vi "Initialize.vi"(8 "error in":errorcluster, 9 "Timeout":u32=100 format="%.0f ms", 10 "Serial Settings":T1={"baud rate"=115200, "data bits"=8, "parity"=enum."None", "stop bits"=10, "flow control"=0} {"flow control" items=["None"=0, "XON/XOFF"=1, "RTS/CTS"=2, "DTR/DSR"=4]; "stop bits" items=["1.0"=10, "1.5"=15, "2.0"=20]; "data bits" min=5 max=8 step=1; "baud rate" items=["75"=75, "110"=110, "134"=134, "150"=150, "300"=300, "600"=600, "1200"=1200, "1800"=1800, "2400"=2400, "4800"=4800, "7200"=7200, "9600"=9600, "14400"=14400, "19200"=19200, "28800"=28800, "38400"=38400, "56000"=56000, "57600"=57600, "115200"=115200, "128000"=128000, "230400"=230400]}, 11 "Comport":refnum<visa-resource-name>="COM8") -> (0 "error out":errorcluster, 3 "Comport Out":refnum<visa-resource-name>)   [LabVIEW 2020, in "MicroPythonClient.lvlib"]
doc: "Initializes the comport for communication with micropython running on the target device."
uses:
  MicroPythonClient.lvlib
  <vilib>/Instr/_visa.llb/VISA Configure Serial Port (Instr).vi
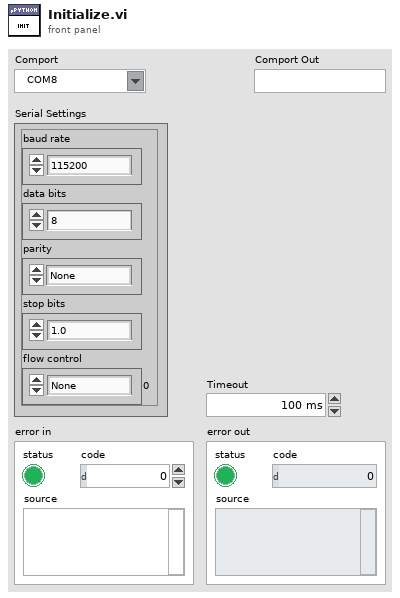
[diagram p1: front panel]
types:
  T1 = cluster{"baud rate":u32, "data bits":u16, "parity":enum16{"None", "Odd", "Even", "Mark", "Space"}, "stop bits":u16, "flow control":u16}
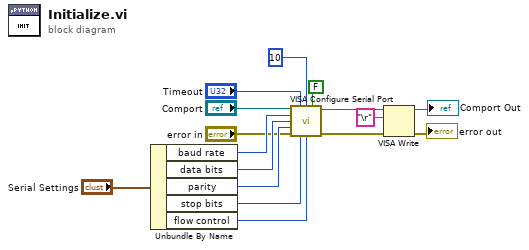
[diagram p0: block diagram]
diagram:
  n1 = Unbundle By Name("Serial Settings") -> ("baud rate"=w16:u32, "data bits"=w15:u16, "parity"=w14:enum16{"None", "Odd", "Even", "Mark", "Space"}, "stop bits"=w13:u16, "flow control"=w12:u16)
  n2 = call-poly "VISA Configure Serial Port"("VISA resource name"="Comport", "timeout (10sec)"="Timeout", "termination char\n(0xA = '\\n' = LF)"=u8 10 ("termination char\n(0xA = '\\n' = LF)"), "Enable Termination\nChar (T)"=FALSE ("Enable Termination\nChar (T)"), "baud rate (9600)"=w16, "data bits (8)"=w15, "parity (0:none)"=w14, "error in (no error)"="error in", "stop bits (10: 1 bit)"=w13, "flow control (0:none)"=w12) -> ("VISA resource name out"=w10:refnum<visa-resource-name>, "error out"=w11:errorcluster)  [unwired: 4 out]
  n3 = VISA Write(VISA resource name=w10, write buffer="\r", error in (no error)=w11) -> (VISA resource name out=→"Comport Out":refnum<visa-resource-name>, error out=→"error out":errorcluster)  [unwired: 1 out]
